vi "Reset.vi"(8 "error in":errorcluster, 11 "Channel":u16) -> (0 "error out":errorcluster, 3 "Channel out":u16)   [LabVIEW 2023, in "PCAN API.lvlib"]
doc: "This VI resets the receive and transmit queues and handles error codes."
uses:
  PCAN API.lvlib
  PCAN2023/PCAN2023.lvlib
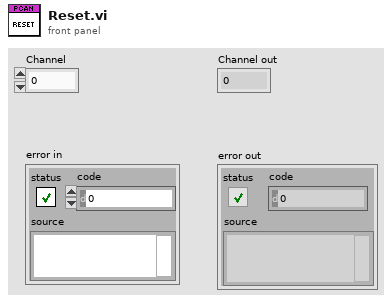
[diagram p1: front panel]
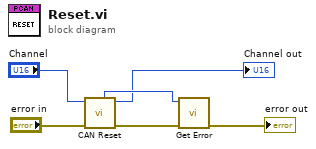
[diagram p0: block diagram]
diagram:
  n1 = call "CAN Reset.vi"("error in"="error in", "Channel"="Channel") -> ("error out"=w6:errorcluster, "Channel out"=→"Channel out":u16, "function return"=w2:u32)  [unwired: 7 in]
  n2 = call "Get Error.vi"("error in (no error)"=w6, "function return"=w2) -> ("error out"=→"error out":errorcluster)  [unwired: 9 in]
